vi "Apply.vi"(8 "error in (no error)":errorcluster, 11 "DIO DAQmx PWM CFG in":refnum<class "CO DAQmx PWM CFG.lvclass">) -> (0 "error out":errorcluster, 3 "DIO DAQmx PWM CFG out":refnum<class "CO DAQmx PWM CFG.lvclass">)   [LabVIEW 2023, in "CO DAQmx PWM CFG.lvclass"]
uses:
  CO DAQmx PWM CFG.lvclass
  CO DAQmx PWM CFG.lvclass/CO DAQmx PWM CFG.ctl
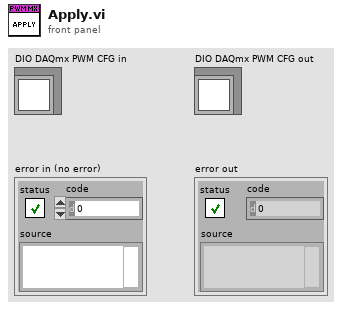
[diagram p1: front panel]
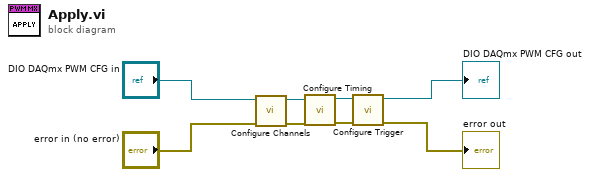
[diagram p0: block diagram]
diagram:
  n1 = call-dynamic "Configure Channels.vi"("error in"="error in (no error)", "DIO DAQmx PWM CFG in"="DIO DAQmx PWM CFG in") -> ("error out"=w3:errorcluster, "DIO DAQmx PWM CFG out"=w4:refnum<class "CO DAQmx PWM CFG.lvclass">)  [unwired: 8 in]
  n2 = call-dynamic "Configure Timing.vi"("error in"=w3, "DAQmx Base CFG in"=w4) -> ("error out"=w1:errorcluster, "DAQmx Base CFG out"=w2:refnum<class "CO DAQmx PWM CFG.lvclass">)  [unwired: 8 in]
  n3 = call-dynamic "Configure Trigger.vi"("error in"=w1, "DAQmx Base CFG in"=w2) -> ("error out"=→"error out":errorcluster, "DAQmx Base CFG out"=→"DIO DAQmx PWM CFG out":refnum<class "CO DAQmx PWM CFG.lvclass">)  [unwired: 8 in]
